vi "Get Ref (inline).vi"(8 "error in (no error)":errorcluster, 11 "BetterHandle in":refnum<class "BetterHandle.lvclass">) -> (0 "error out":errorcluster, 2 "Tree/LB/MCL ref":refnum<vi>, 3 "BetterHandle out":refnum<class "BetterHandle.lvclass">)   [LabVIEW 2020, in "BetterDragAndDrop.lvlib" / "BetterHandle.lvclass"]
uses:
  BetterHandle.lvclass
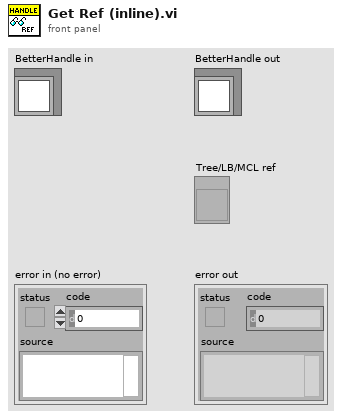
[diagram p1: front panel]
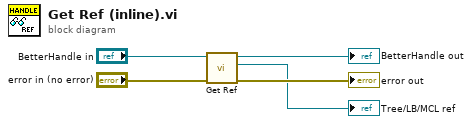
[diagram p0: block diagram]
diagram:
  n1 = call-dynamic "Get Ref.vi"("error in (no error)"="error in (no error)", "BetterHandle in"="BetterHandle in") -> ("error out"=→"error out":errorcluster, "Tree/LB/MCL ref"=→"Tree/LB/MCL ref":refnum<vi>, "BetterHandle out"=→"BetterHandle out":refnum<class "BetterHandle.lvclass">)  [unwired: 7 in]
